vi "Untitled 2.vi"   [LabVIEW 2017]
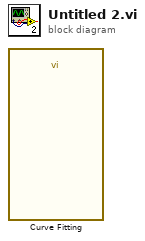
[diagram p0: block diagram]
diagram:
  n1 = call "Curve Fitting"() -> ()  [unwired: 7 in, 5 out]
